vi "LabVIEW_Matlab.vi"() -> ()   [LabVIEW 2017]
uses:
  <vilib>/imath/engines/lvmath/Plug In/_Char/NIMS_CH_character datatype.ctl
  <vilib>/imath/engines/lvmath2/RunTimeEngine/Managers/WorkSpace/UID Generator.vi
  <vilib>/imath/engines/lvmath2/RunTimeEngine/BuiltInFunctions/abs/NIMS_abs(signed).vi
  <instcachedir>/0/NIMS_abs(signed)_C4FCB8E6058B49B797C7C8D53CA5F6EC.lvgen/NIMS_abs(signed)_C4FCB8E6058B49B797C7C8D53CA5F6EC_006.vi
  <vilib>/imath/engines/lvmath2/RunTimeEngine/BuiltInFunctions/angle/NIMS_angle.vi
  <instcachedir>/0/NIMS_angle_6DDAE2BD99E0421EB990B6436E94D88F.lvgen/NIMS_angle_6DDAE2BD99E0421EB990B6436E94D88F_002.vi
  <vilib>/imath/engines/lvmath2/RunTimeEngine/BuiltInFunctions/max/1 input/NIMS_max(RV).vi
  <instcachedir>/0/NIMS_max(RV)_237633DB1D604D5BA7001287DF3C7957.lvgen/NIMS_max(RV)_237633DB1D604D5BA7001287DF3C7957_000.vi
  <vilib>/imath/engines/lvmath2/RunTimeEngine/BuiltInFunctions/findnz/NIMS_[1o]_findnz(GRowV).vi
  <instcachedir>/0/NIMS_[1o]_findnz(GRowV)_3E31462E2BB14E3DAA95AD1E75EDC533.lvgen/NIMS_[1o]_findnz(GRowV)_3E31462E2BB14E3DAA95AD1E75EDC533_000.vi
  <vilib>/imath/engines/lvmath2/RunTimeEngine/RunTimeType/NIMS_RunTimeType_From StrictType (excl LVString).vi
  <instcachedir>/0/NIMS_RunTimeType_From StrictType (excl LVString)_1019F277F0A747EDBCA0F6C52CA54500.lvgen/NIMS_RunTimeType_From StrictType (excl LVString)_1019F277F0A747EDBCA0F6C52CA54500_000.vi
  <vilib>/imath/engines/lvmath2/RunTimeEngine/LocalVariableDefStatement/MC_LocalVariableDefStatement_Display.vi
  <vilib>/imath/engines/lvmath2/RunTimeEngine/BuiltInFunctions/min/1 input/NIMS_min(RV).vi
  <instcachedir>/0/NIMS_min(RV)_EE2DD3E2888846108C5160A664B67832.lvgen/NIMS_min(RV)_EE2DD3E2888846108C5160A664B67832_000.vi
  <vilib>/imath/engines/lvmath2/RunTimeEngine/BuiltInFunctions/figure/NIMS_figure(I32).vi
  <vilib>/imathl/engines/lvmath/Functions/Error Handling/Create Error.vi
  <vilib>/imath/engines/lvmath2/RunTimeEngine/BuiltInFunctions/plotyy/NIMS_plotyy.vi
  <vilib>/imath/engines/lvmath2/RunTimeEngine/BuiltInFunctions/axis/NIMS_axis.vi
  <vilib>/imath/engines/lvmath/Plug In/_Char/NIMS_CH_Character RV to String.vi
  <vilib>/imath/engines/lvmath2/RunTimeEngine/BuiltInFunctions/title/NIMS_title.vi
  <vilib>/imath/engines/lvmath2/RunTimeEngine/BuiltInFunctions/xlabel/NIMS_xlabel.vi
  <vilib>/imath/engines/lvmath2/RunTimeEngine/BuiltInFunctions/grid/NIMS_grid(Enums).vi
  <vilib>/imath/engines/lvmath2/RunTimeEngine/IndexRead/NIMS V(V).vi
  <instcachedir>/0/NIMS V(V)_298D9CB7BFEB42B8BC8D9C3C28AE8C70.lvgen/NIMS V(V)_298D9CB7BFEB42B8BC8D9C3C28AE8C70_000.vi
  <vilib>/imath/engines/lvmath2/RunTimeEngine/BuiltInFunctions/num_to_str/NIMS_num_to_str(GRowV,I32).vi
  <instcachedir>/0/NIMS_num_to_str(GRowV,I32)_E276F6938A3A4382A40154016B10DDC2.lvgen/NIMS_num_to_str(GRowV,I32)_E276F6938A3A4382A40154016B10DDC2_000.vi
  <vilib>/imath/engines/lvmath/Plug In/_Char/NIMS_CH_String to Character Array.vi
  <vilib>/imath/engines/lvmath2/RunTimeSupport/NIMS_Get Scalar_w Error.vi
  <instcachedir>/0/NIMS_Get Scalar_w Error_1987D997E87247DDAC16EA23A5E9E4FC.lvgen/NIMS_Get Scalar_w Error_1987D997E87247DDAC16EA23A5E9E4FC_010.vi
  <instcachedir>/0/NIMS V(V)_298D9CB7BFEB42B8BC8D9C3C28AE8C70.lvgen/NIMS V(V)_298D9CB7BFEB42B8BC8D9C3C28AE8C70_001.vi
  <vilib>/imath/engines/lvmath2/RunTimeEngine/ArithmeticOperatorToken/NIMS_ArithmeticOperator_plus.vi
  <instcachedir>/0/NIMS_ArithmeticOperator_plus_9255C7DA94A9479C92F91DC2DA9A664F.lvgen/NIMS_ArithmeticOperator_plus_9255C7DA94A9479C92F91DC2DA9A664F_001.vi
  <vilib>/imath/engines/lvmath2/RunTimeEngine/ErrorHandling/NIMS_Create Error From Enums.vi
  <vilib>/imath/engines/lvmath2/RunTimeEngine/BuiltInFunctions/text/NIMS_text.vi
  <vilib>/imath/engines/lvmath2/RunTimeEngine/Managers/SymbolTable/Clear UID.vi
  <vilib>/imath/engines/lvmath2/RunTimeEngine/ErrorHandling/NIMS_Finalize Error.vi
  <vilib>/imath/engines/lvmath2/RunTimeEngine/RangeToken/NIMS_Range.vi
  <instcachedir>/0/NIMS_Range_69CB9AAD882742A19CF7E739BE79952C.lvgen/NIMS_Range_69CB9AAD882742A19CF7E739BE79952C_000.vi
  <vilib>/imath/engines/lvmath2/RunTimeEngine/BuiltInFunctions/plot/NIMS_plot(RM, RM, Str).vi
  <vilib>/imath/engines/lvmath2/RunTimeEngine/BuiltInFunctions/ylabel/NIMS_ylabel.vi
  <vilib>/imath/engines/lvmath2/RunTimeEngine/BuiltInFunctions/hold/NIMS_hold(Enums).vi
  <vilib>/imath/engines/lvmath/Plug In/_Char/NIMS_CH_Character 2D to String 1D.vi
  <vilib>/imath/engines/lvmath2/RunTimeEngine/BuiltInFunctions/strconcat/NIMS_strconcat.vi
  <vilib>/imath/engines/lvmath/Plug In/_Char/NIMS_CH_String CV to Character 2D.vi
  <instcachedir>/0/NIMS_CH_String CV to Character 2D_E74A305AD5CE4F8EB468AF2B6B40BB87.lvgen/NIMS_CH_String CV to Character 2D_E74A305AD5CE4F8EB468AF2B6B40BB87_000.vi
  <vilib>/imath/engines/lvmath2/RunTimeSupport/NIMS_Get Row Vector_w Error - Matrix.vi
  <instcachedir>/0/NIMS_Get Row Vector_w Error - Matrix_7ECCFA0649AF47C08F6F0C496599EB01.lvgen/NIMS_Get Row Vector_w Error - Matrix_7ECCFA0649AF47C08F6F0C496599EB01_000.vi
  <vilib>/imath/engines/lvmath2/RunTimeEngine/BuiltInFunctions/legend/NIMS_legend(Arb).vi
  <vilib>/imath/engines/lvmath2/RunTimeEngine/Managers/SymbolTable/NIMS_WorkSpace.lvlib
panel:
  in  "开始计算":bool
  in  "开始计算":bool
  in  "开始计算":bool
  in  "开始计算":bool
  in  "开始计算":bool
  in  "开始计算":bool
  in  "开始计算":bool
  out "夹持电容":dbl
  out "动态电感":dbl
  out "动态电容":dbl
  out "动态电阻":dbl
  in  "?":bool
  in  "并联谐振频率":dbl
  in  "?":bool
  in  "?":bool
  in  "?":bool
  in  "串联谐振频率":dbl
  in  "定子最小导纳":dbl
  in  "定子最大导纳":dbl
  in  "动态电容3":dbl
  in  "动态电容2":dbl
  in  "动态电容1":dbl
  in  "动态电感3":dbl
  in  "动态电感2":dbl
  in  "动态电感1":dbl
  in  "夹持电容3":dbl
  in  "夹持电容2":dbl
  in  "夹持电容1":dbl
  in  "动态电阻3":dbl
  in  "动态电阻2":dbl
  in  "动态电阻1":dbl
  # "阻抗测试模块"
  # "概述：Matlab仿真模块，定子导纳-频率图、定子导纳圆及动态电阻、动态电感、动态电容、夹持电容变化导致的相关影响。"
  # "result"
  # "动态电感"
  # "动态电阻"
  # "input"
  # "超声波电机导纳-频率图"
  # "注意：默认值为450、735.7、1200.7"
  # "注意：默认值为0.239、0.229、0.219"
  # "定子导纳圆、\n定子导纳-频率图"
  # "动态电容"
  # "夹持电容"
  # "注意：默认值为2.36e-9、3.36e-9、4.36e-9"
  # "注意：默认值为34.7e-12、36.7e-12、38.7e-12"
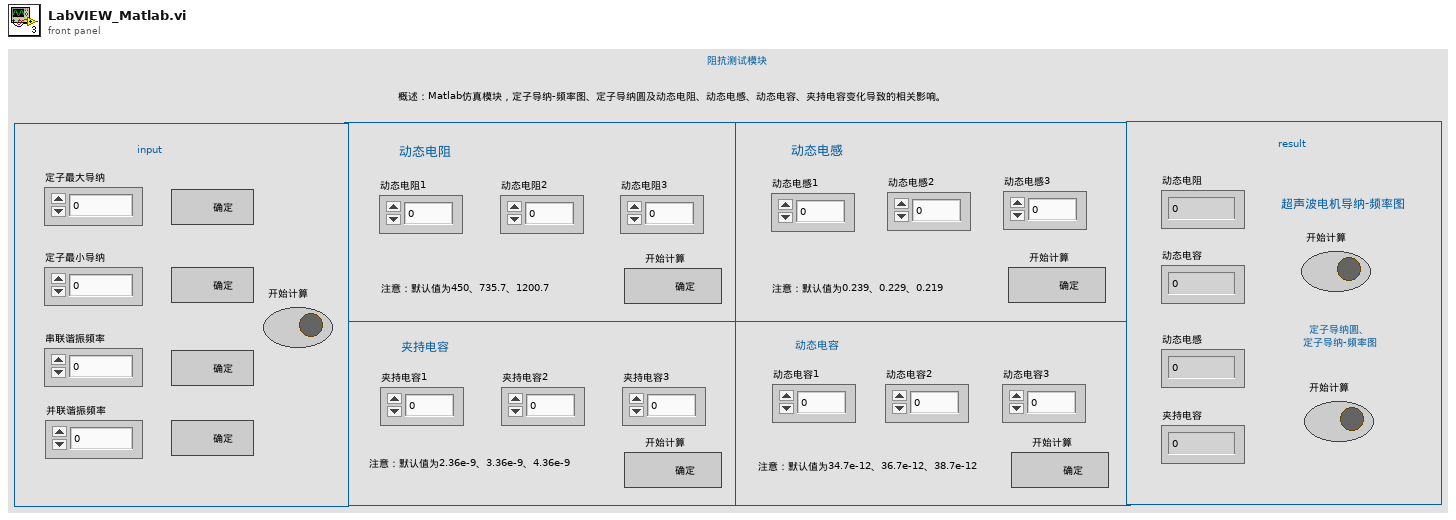
[diagram p1: front panel]
types:
  T1 = typedef "NIMS_CH_character datatype.ctl" = cluster{"Numeric":u8}
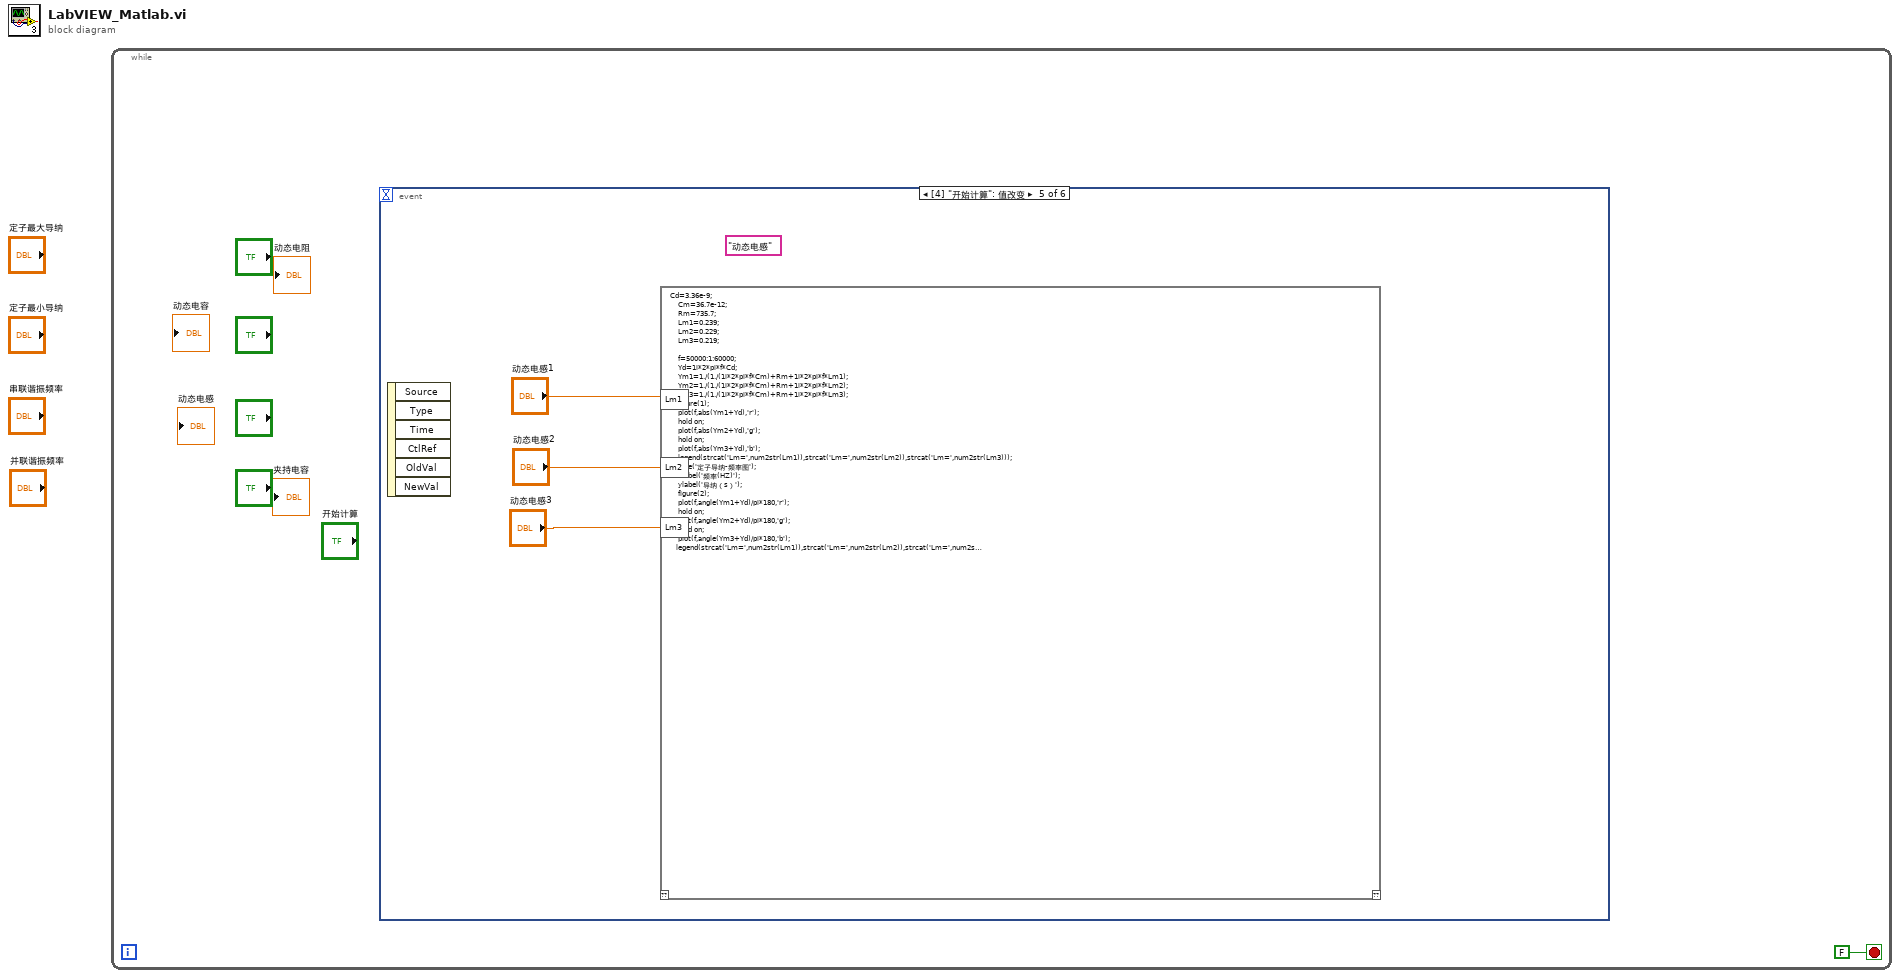
[diagram p0: block diagram]
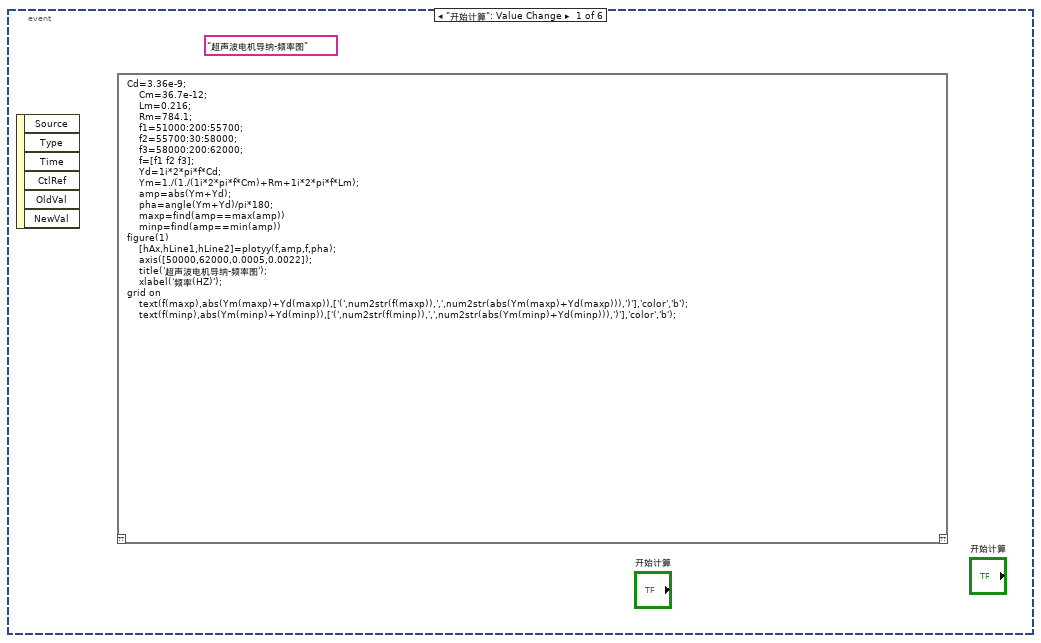
[diagram p2: hidden frame]
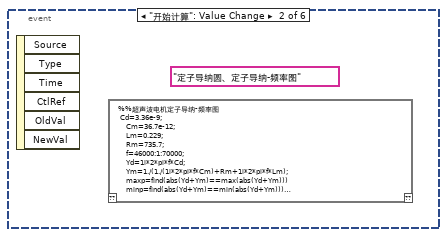
[diagram p3: hidden frame]
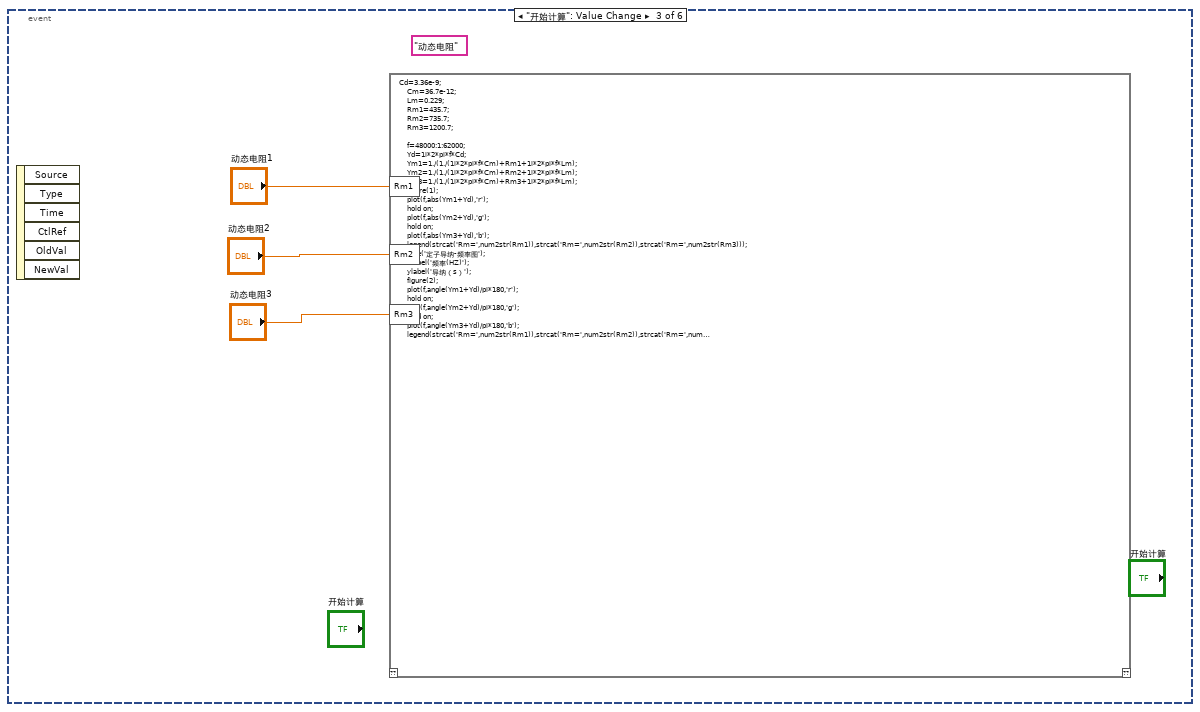
[diagram p4: hidden frame]
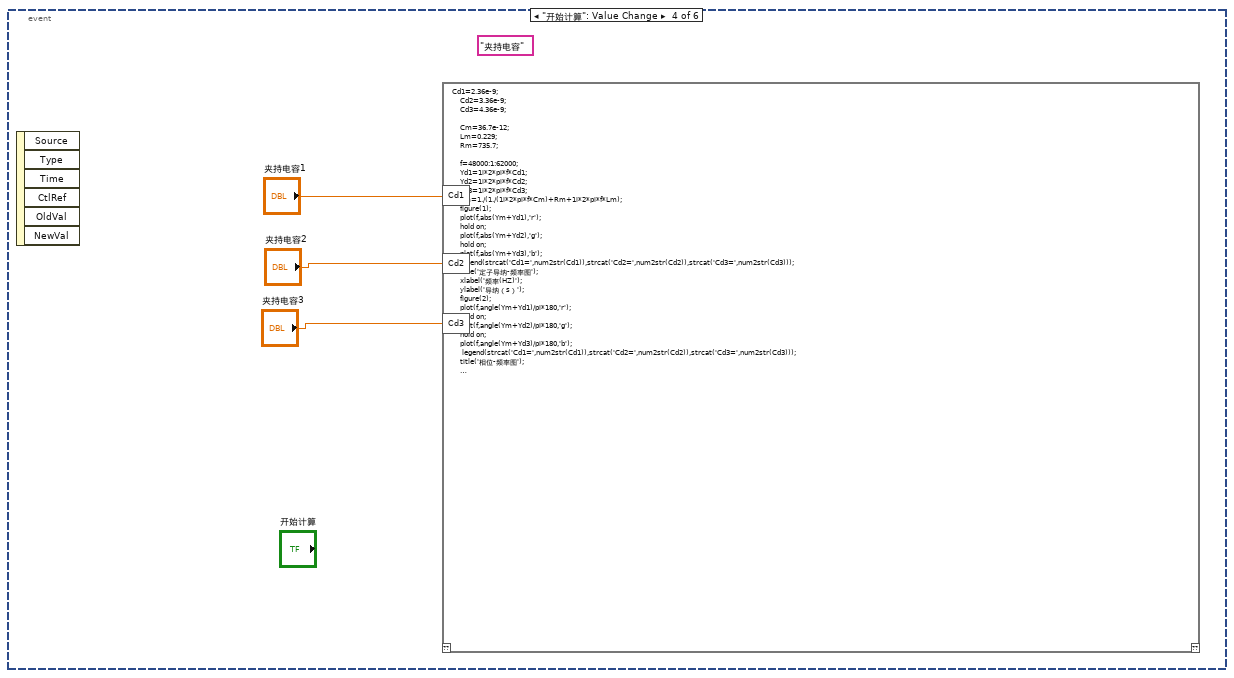
[diagram p5: hidden frame]
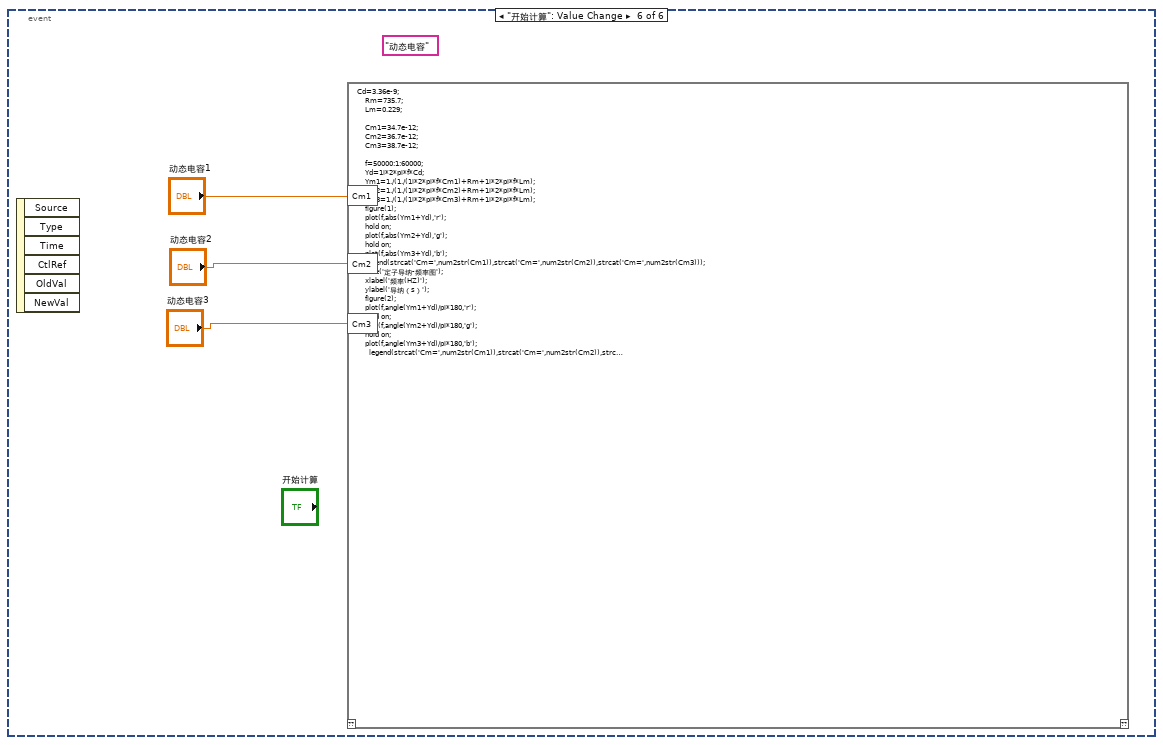
[diagram p6: hidden frame]
diagram:
  n1 = while {
    stop <- FALSE stop-if-true
    n2 = event shown="[4] \"开始计算\": 值改变" {
      selector: _ -> [_ _ _ _ _ _]
      dyn-events: _ -> [_ _ _ _ _ _]
      timeout: _ -> [_ _ _ _ _ _]
      event "开始计算": Value Change {
        (unwired) "超声波电机导纳-频率图"
        n3 = event-data() -> ()  [unwired: 1 in, 6 out]
        n4 = mathscript code="Cd=3.36e-9;\n    Cm=36.7e-12;\n    Lm=0.216;\n    Rm=784.1;\n    f1=51000:200:55700;\n    f2=55700:30:58000;\n    f3=58000:200:62000;\n    f=[f1 f2 f3];                                                                                                                                                                                                                                                                                                                                                                                                                                                                                                                                                                                                                                                                                                                                                                                                                                                                                                                                                                                                                                                                                                                                                                                                                                           \n    Yd=1i*2*pi*f*Cd;\n    Ym=1./(1./(1i*2*pi*f*Cm)+Rm+1i*2*pi*f*Lm);\n    amp=abs(Ym+Yd);\n    pha=angle(Ym+Yd)/pi*180;\n    maxp=find(amp==max(amp))\n    minp=find(amp==min(amp))\nfigure(1)\n    [hAx,hLine1,hLine2]=plotyy(f,amp,f,pha);\n    axis([50000,62000,0.0005,0.0022]);\n    title('超声波电机导纳-频率图');\n    xlabel('频率(HZ)');\ngrid on\n    text(f(maxp),abs(Ym(maxp)+Yd(maxp)),['(',num2str(f(maxp)),',',num2str(abs(Ym(maxp)+Yd(maxp))),')'],'color','b');\n    text(f(minp),abs(Ym(minp)+Yd(minp)),['(',num2str(f(minp)),',',num2str(abs(Ym(minp)+Yd(minp))),')'],'color','b');"() -> ()  [unwired: 1 in, 1 out]
      }
      event "开始计算": Value Change {
        (unwired) "定子导纳圆、定子导纳-频率图"
        n5 = event-data() -> ()  [unwired: 1 in, 6 out]
        n6 = mathscript code="%%超声波电机定子导纳-频率图\n Cd=3.36e-9;\n    Cm=36.7e-12;\n    Lm=0.229;\n    Rm=735.7;\n    f=46000:1:70000;                                                                                                                                                                                                                                                                                                                                                                                                                                                                                                                                                                                                                                                                                                                                                                                                                                                                                                                                                                                                                                                                                                                                                                                                                                             \n    Yd=1i*2*pi*f*Cd;\n    Ym=1./(1./(1i*2*pi*f*Cm)+Rm+1i*2*pi*f*Lm);\n    maxp=find(abs(Yd+Ym)==max(abs(Yd+Ym)))\n    minp=find(abs(Yd+Ym)==min(abs(Yd+Ym)))\n figure(1)\n plotyy(f,abs(Ym+Yd),f,angle(Ym+Yd)/pi*180);\n    title('定子导纳-频率图');\n    xlabel('频率(Hz)');\n    grid on;\n    text(f(maxp),abs(Ym(maxp)+Yd(maxp)),['(',num2str(f(maxp)),',',num2str(abs(Ym(maxp)+Yd(maxp))),')'],'color','b');\n    text(f(minp),abs(Ym(minp)+Yd(minp)),['(',num2str(f(minp)),',',num2str(abs(Ym(minp)+Yd(minp))),')'],'color','b');   \n\n alpha=0:pi/20:2*pi;\n    R=0.6796;\n    x=R*cos(alpha)+0.6796;\n    y=R*sin(alpha)+1.155;\nfigure(2)\n    plot(x,y,'o-');\n    title('定子导纳图');\n    xlabel('G');\n    ylabel('B');\n    axis([0,1.6,0.4,2]);"() -> ()  [unwired: 1 in, 1 out]
      }
      event "开始计算": Value Change {
        (unwired) "动态电阻"
        n7 = event-data() -> ()  [unwired: 1 in, 6 out]
        n8 = mathscript code="Cd=3.36e-9;\n    Cm=36.7e-12;\n    Lm=0.229;\n    Rm1=435.7;\n    Rm2=735.7;\n    Rm3=1200.7;\n\n    f=48000:1:62000;                                                                                                                                                                                                                                                                                                                                                                                                                                                                                                                                                                                                                                                                                                                                                                                                                                                                                                                                                                                                                                                                                                                                                                                                                                             \n    Yd=1i*2*pi*f*Cd;\n    Ym1=1./(1./(1i*2*pi*f*Cm)+Rm1+1i*2*pi*f*Lm);\n    Ym2=1./(1./(1i*2*pi*f*Cm)+Rm2+1i*2*pi*f*Lm);\n    Ym3=1./(1./(1i*2*pi*f*Cm)+Rm3+1i*2*pi*f*Lm);\n    figure(1);\n    plot(f,abs(Ym1+Yd),'r');\n    hold on;\n    plot(f,abs(Ym2+Yd),'g');\n    hold on;\n    plot(f,abs(Ym3+Yd),'b');\n    legend(strcat('Rm=',num2str(Rm1)),strcat('Rm=',num2str(Rm2)),strcat('Rm=',num2str(Rm3)));\n    title('定子导纳-频率图');\n    xlabel('频率(HZ)');\n    ylabel('导纳（s）');\n    figure(2);\n    plot(f,angle(Ym1+Yd)/pi*180,'r');\n    hold on;\n    plot(f,angle(Ym2+Yd)/pi*180,'g');\n    hold on;\n    plot(f,angle(Ym3+Yd)/pi*180,'b');\n    legend(strcat('Rm=',num2str(Rm1)),strcat('Rm=',num2str(Rm2)),strcat('Rm=',num2str(Rm3)));\n    title('相位-频率图');\n    xlabel('频率(HZ)');\n    ylabel('相位（°）');"("Rm1"="动态电阻1", "Rm2"="动态电阻2", "Rm3"="动态电阻3") -> ()  [unwired: 1 in, 1 out]
      }
      event "开始计算": Value Change {
        (unwired) "夹持电容"
        n9 = event-data() -> ()  [unwired: 1 in, 6 out]
        n10 = mathscript code="Cd1=2.36e-9;\n    Cd2=3.36e-9;\n    Cd3=4.36e-9;\n   \n    Cm=36.7e-12;\n    Lm=0.229;\n    Rm=735.7;\n\n    f=48000:1:62000;                                                                                                                                                                                                                                                                                                                                                                                                                                                                                                                                                                                                                                                                                                                                                                                                                                                                                                                                                                                                                                                                                                                                                                                                                                             \n    Yd1=1i*2*pi*f*Cd1;\n    Yd2=1i*2*pi*f*Cd2;\n    Yd3=1i*2*pi*f*Cd3;\n    Ym=1./(1./(1i*2*pi*f*Cm)+Rm+1i*2*pi*f*Lm);\n    figure(1);\n    plot(f,abs(Ym+Yd1),'r');\n    hold on;\n    plot(f,abs(Ym+Yd2),'g');\n    hold on;\n    plot(f,abs(Ym+Yd3),'b');\n    legend(strcat('Cd1=',num2str(Cd1)),strcat('Cd2=',num2str(Cd2)),strcat('Cd3=',num2str(Cd3)));\n    title('定子导纳-频率图');\n    xlabel('频率(HZ)');\n    ylabel('导纳（s）');\n    figure(2);\n    plot(f,angle(Ym+Yd1)/pi*180,'r');\n    hold on;\n    plot(f,angle(Ym+Yd2)/pi*180,'g');\n    hold on;\n    plot(f,angle(Ym+Yd3)/pi*180,'b');\n     legend(strcat('Cd1=',num2str(Cd1)),strcat('Cd2=',num2str(Cd2)),strcat('Cd3=',num2str(Cd3)));\n    title('相位-频率图');\n    xlabel('频率(HZ)');\n    ylabel('相位（°）');"("Cd1"="夹持电容1", "Cd2"="夹持电容2", "Cd3"="夹持电容3") -> ()  [unwired: 1 in, 1 out]
      }
      event "开始计算": Value Change {
        (unwired) "动态电感"
        n11 = event-data() -> ()  [unwired: 1 in, 6 out]
        n12 = mathscript code="Cd=3.36e-9;\n    Cm=36.7e-12;\n    Rm=735.7;\n    Lm1=0.239;\n    Lm2=0.229;\n    Lm3=0.219;\n\n    f=50000:1:60000;                                                                                                                                                                                                                                                                                                                                                                                                                                                                                                                                                                                                                                                                                                                                                                                                                                                                                                                                                                                                                                                                                                                                                                                                                                             \n    Yd=1i*2*pi*f*Cd;\n    Ym1=1./(1./(1i*2*pi*f*Cm)+Rm+1i*2*pi*f*Lm1);\n    Ym2=1./(1./(1i*2*pi*f*Cm)+Rm+1i*2*pi*f*Lm2);\n    Ym3=1./(1./(1i*2*pi*f*Cm)+Rm+1i*2*pi*f*Lm3);\n    figure(1);\n    plot(f,abs(Ym1+Yd),'r');\n    hold on;\n    plot(f,abs(Ym2+Yd),'g');\n    hold on;\n    plot(f,abs(Ym3+Yd),'b');\n    legend(strcat('Lm=',num2str(Lm1)),strcat('Lm=',num2str(Lm2)),strcat('Lm=',num2str(Lm3)));\n    title('定子导纳-频率图');\n    xlabel('频率(HZ)');\n    ylabel('导纳（s）');\n    figure(2);\n    plot(f,angle(Ym1+Yd)/pi*180,'r');\n    hold on;\n    plot(f,angle(Ym2+Yd)/pi*180,'g');\n    hold on;\n    plot(f,angle(Ym3+Yd)/pi*180,'b');\n   legend(strcat('Lm=',num2str(Lm1)),strcat('Lm=',num2str(Lm2)),strcat('Lm=',num2str(Lm3)));\n    title('相位-频率图');\n    xlabel('频率(HZ)');\n    ylabel('相位（°）');"("Lm1"="动态电感1", "Lm2"="动态电感2", "Lm3"="动态电感3") -> ()  [unwired: 1 in, 1 out]
      }
      event "开始计算": Value Change {
        (unwired) "动态电容"
        n13 = event-data() -> ()  [unwired: 1 in, 6 out]
        n14 = mathscript code="Cd=3.36e-9;\n    Rm=735.7;\n    Lm=0.229;\n    \n    Cm1=34.7e-12;\n    Cm2=36.7e-12;\n    Cm3=38.7e-12;\n\n    f=50000:1:60000;                                                                                                                                                                                                                                                                                                                                                                                                                                                                                                                                                                                                                                                                                                                                                                                                                                                                                                                                                                                                                                                                                                                                                                                                                                             \n    Yd=1i*2*pi*f*Cd;\n    Ym1=1./(1./(1i*2*pi*f*Cm1)+Rm+1i*2*pi*f*Lm);\n    Ym2=1./(1./(1i*2*pi*f*Cm2)+Rm+1i*2*pi*f*Lm);\n    Ym3=1./(1./(1i*2*pi*f*Cm3)+Rm+1i*2*pi*f*Lm);\n    figure(1);\n    plot(f,abs(Ym1+Yd),'r');\n    hold on;\n    plot(f,abs(Ym2+Yd),'g');\n    hold on;\n    plot(f,abs(Ym3+Yd),'b');\n    legend(strcat('Cm=',num2str(Cm1)),strcat('Cm=',num2str(Cm2)),strcat('Cm=',num2str(Cm3)));\n    title('定子导纳-频率图');\n    xlabel('频率(HZ)');\n    ylabel('导纳（s）');\n    figure(2);\n    plot(f,angle(Ym1+Yd)/pi*180,'r');\n    hold on;\n    plot(f,angle(Ym2+Yd)/pi*180,'g');\n    hold on;\n    plot(f,angle(Ym3+Yd)/pi*180,'b');\n      legend(strcat('Cm=',num2str(Cm1)),strcat('Cm=',num2str(Cm2)),strcat('Cm=',num2str(Cm3)));\n    title('相位-频率图');\n    xlabel('频率(HZ)');\n    ylabel('相位（°）');"("Cm1"="动态电容1", "Cm2"="动态电容2", "Cm3"="动态电容3") -> ()  [unwired: 1 in, 1 out]
      }
    }
  }
